vi "Step Convert Datasheet Parameters.vi"(5 "Conversion":enum16{"DB - Cluster", "Cluster - DB"}(ring), 7 "Datasheets":T1, 8 "Data String":string) -> (1 "Data String":string, 2 "Datasheets":T1)   [LabVIEW 2011]
uses:
  www/tests/Test Datasheets.ctl
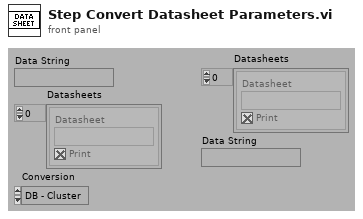
[diagram p1: front panel]
types:
  T1 = typedef "Test Datasheets.ctl" = cluster{"Datasheet":string, "Print":bool}[]
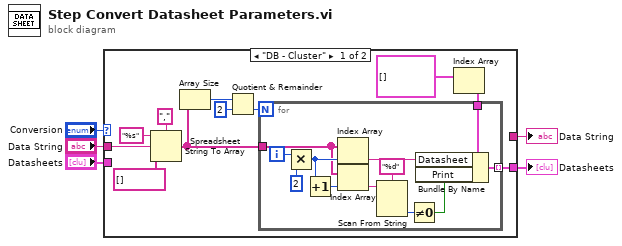
[diagram p0: block diagram]
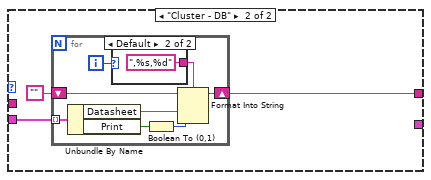
[diagram p2: hidden frame]
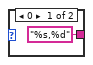
[diagram p3: hidden frame]
diagram:
  n1 = case shown="\"DB - Cluster\"" "Conversion" {
    tunnel: [w10 _] -> w1
    tunnel: "Data String" -> [w9 _]
    tunnel: "Datasheets" -> [_ w31]
    tunnel: [_ w29] -> w2
    frame "DB - Cluster" {
      n2 = Spreadsheet String To Array(delimiter (Tab)=",", format string="%s", spreadsheet string=w9, array type (2D Dbl)=string[] []) -> (array=w13:string[])
      n3 = Array Size(array=w13) -> (size(s)=w14:i32)
      n4 = Quotient & Remainder(x=w14, y=2) -> (floor(x/y)=w16:i32)  [unwired: 1 out]
      n5 = Index Array(array=T1 [] ("Datasheets")) -> (element=w12:cluster{"Datasheet":string, "Print":bool})  [unwired: 1 in]
      n6 = for {
        N: w16 -> [_]
        tunnel: w13 -> [w23]
        tunnel: [w18] -> w10 mode=indexing
        tunnel: w12 -> [w17]
        i -> [w28]
        n7 = Multiply(x=w28, y=2) -> (x*y=w26:i32)
        n8 = Increment(x=w26) -> (x+1=w25:i32)
        n9 = Index Array(array=w23, index=w26) -> (element=w19:string)
        n10 = Index Array(array=w23, index=w25) -> (element=w24:string)
        n11 = Scan From String(format string="%d", input string=w24) -> (output 1=w21:i32)  [unwired: 2 in, 4 out]
        n12 = Not Equal To 0?(x=w21) -> (x != 0?=w20:bool)
        n13 = Bundle By Name(cluster=w17, "Datasheet"=w19, "Print"=w20) -> (w18:cluster{"Datasheet":string, "Print":bool})
      }
    }
    frame "Cluster - DB" {
      n14 = for {
        tunnel: w31 -> [w39] mode=indexing
        shift-right: [w32] -> w29
        shift-left: "" -> [w34]
        i -> [w33]
        n15 = Unbundle By Name(w39) -> ("Datasheet"=w36:string, "Print"=w38:bool)
        n16 = case shown="Default" w33 {
          tunnel: ["%s,%d" ("format string") ",%s,%d" ("format string")] -> w35
          frame 0 {
          }
          frame Default {
          }
        }
        n17 = Boolean To (0,1)(Boolean=w38) -> (0, 1=w37:i16)
        n18 = Format Into String(format string=w35, initial string=w34, w36, w37) -> (resulting string=w32:string)  [unwired: 1 in, 1 out]
      }
    }
  }
  "Datasheets" <- w1
  "Data String" <- w2
